vi "HostCameraManager.vi"() -> ()   [LabVIEW 2024]
panel:
  in  "Exposure":dbl(slide) scale=0.2..3.0
  out "Remote Capture":bool
  out "Live":bool
  out "FPS":dbl(graph)
  out "Image":u16[][](graph)
  in  "stop":bool
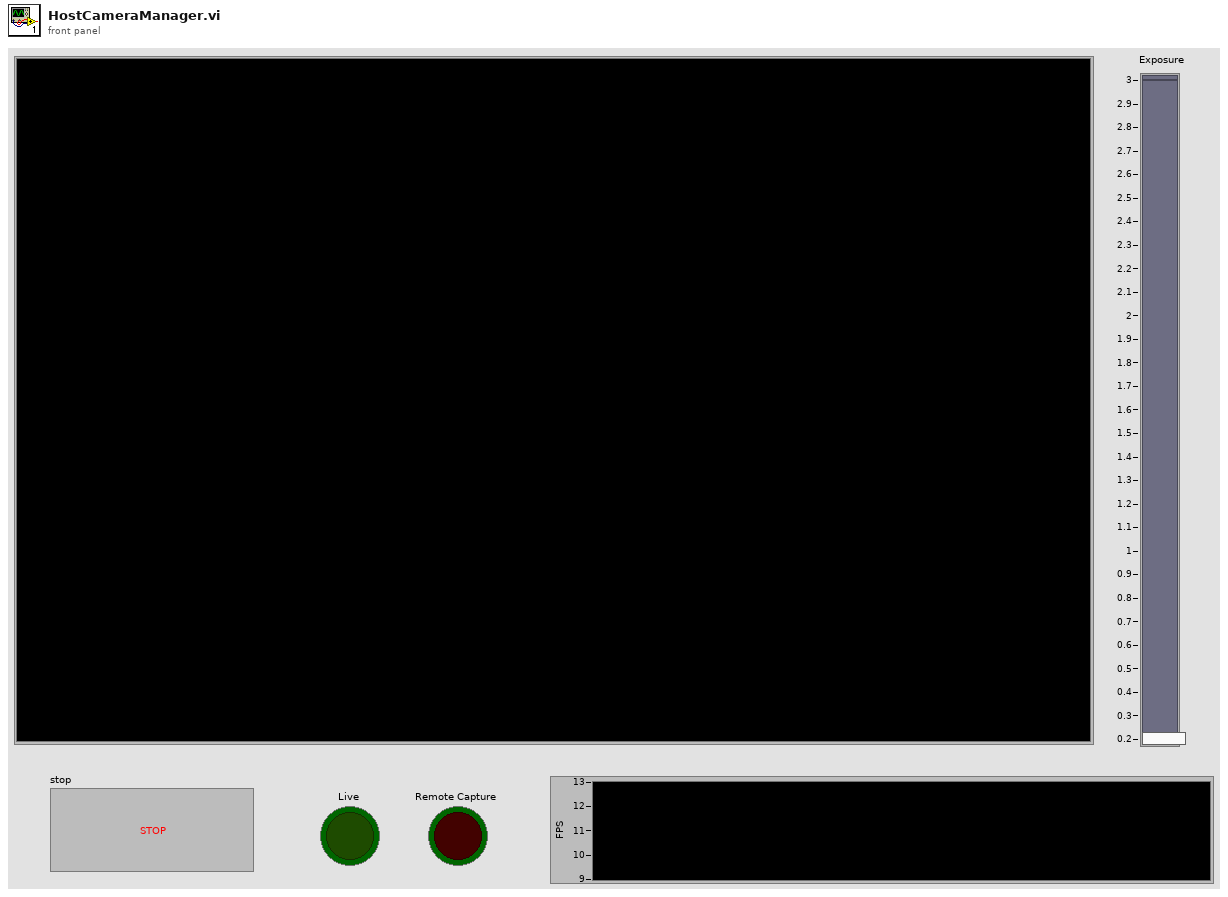
[diagram p1: front panel]
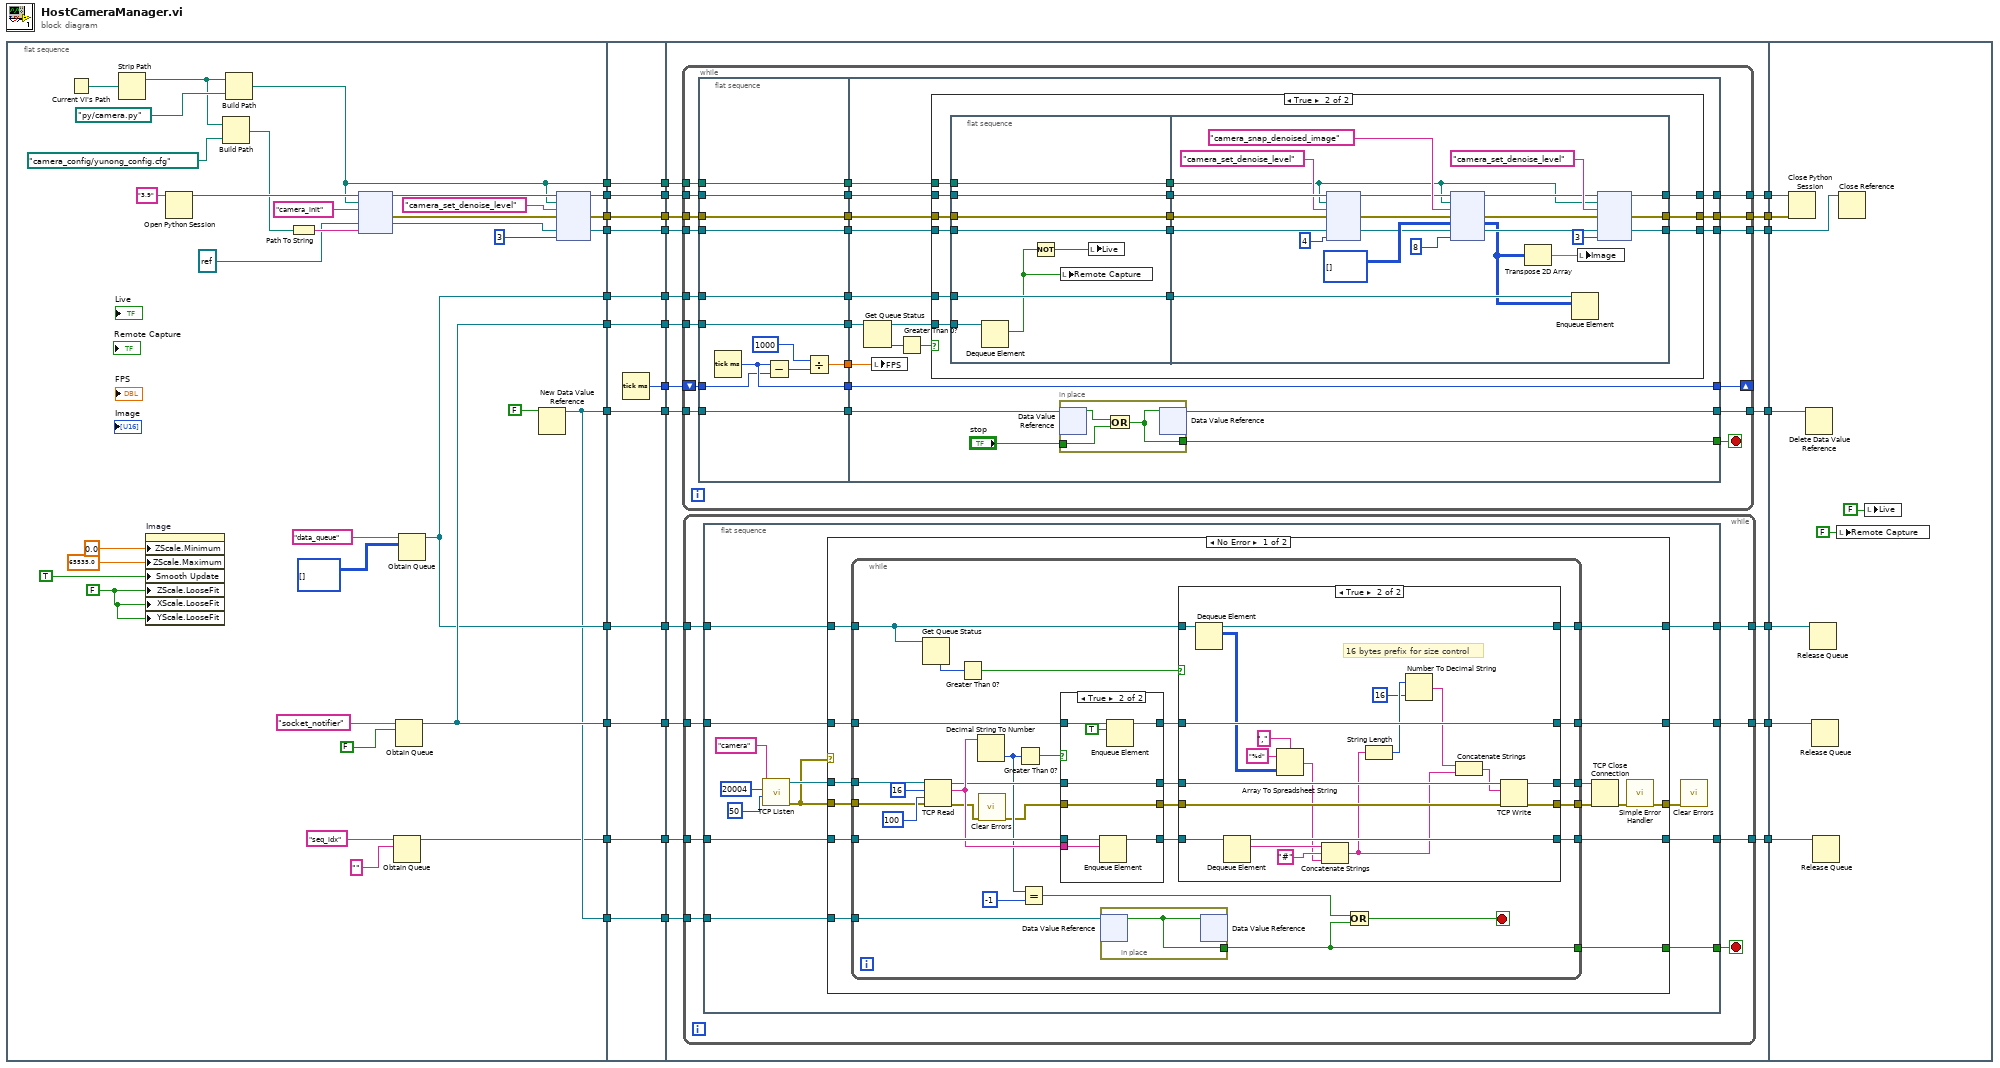
[diagram p0: block diagram]
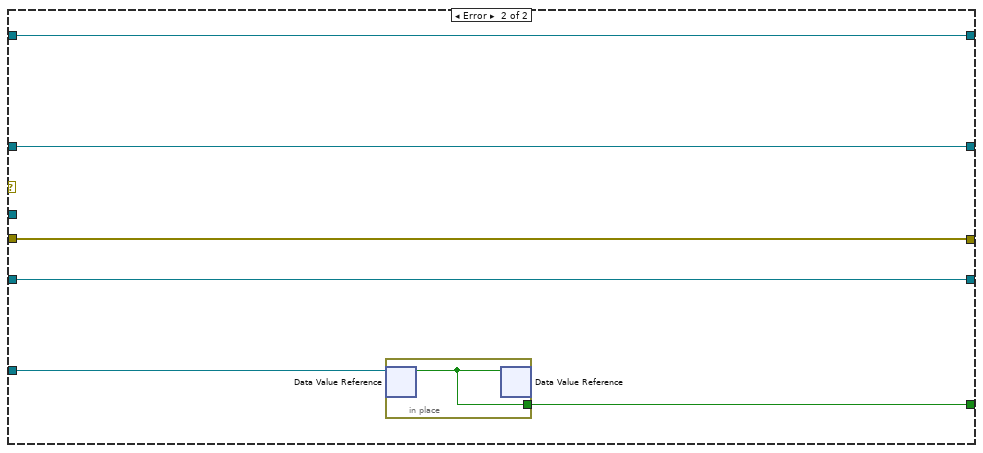
[diagram p4: hidden frame]
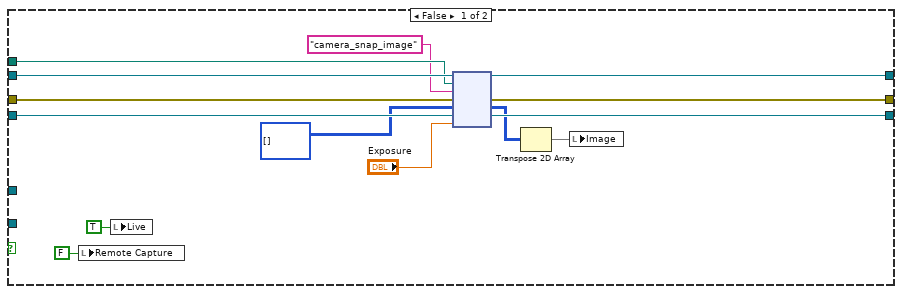
[diagram p5: hidden frame]
diagram:
  n1 = flat-sequence {
    tunnel: [w52] -> w27
    tunnel: [w51] -> w25
    tunnel: [w47] -> w23
    tunnel: [w46] -> w21
    tunnel: [w34] -> w17
    tunnel: [w36] -> w14
    tunnel: [w35] -> w12
    tunnel: [w36] -> w10
    tunnel: [w35] -> w8
    tunnel: [w34] -> w6
    tunnel: [w32] -> w4
    tunnel: w27 -> [w76]
    tunnel: [w76] -> w26
    tunnel: w25 -> [w75]
    tunnel: [w75] -> w24
    tunnel: w23 -> [w74]
    tunnel: [w74] -> w22
    tunnel: w21 -> [w73]
    tunnel: [w73] -> w20
    tunnel: [w72] -> w19
    tunnel: [w71] -> w18
    tunnel: w17 -> [w71]
    tunnel: [w70] -> w15
    tunnel: w14 -> [w70]
    tunnel: [w69] -> w13
    tunnel: w12 -> [w69]
    tunnel: [w68] -> w11
    tunnel: w10 -> [w68]
    tunnel: [w67] -> w9
    tunnel: w8 -> [w67]
    tunnel: [w66] -> w7
    tunnel: w6 -> [w66]
    tunnel: [w65] -> w5
    tunnel: w4 -> [w65]
    tunnel: w26 -> [w94]
    tunnel: w24 -> [w93]
    tunnel: w22 -> [w95]
    tunnel: w20 -> [w92]
    tunnel: [w91] -> w30
    tunnel: [w90] -> w29
    tunnel: [w89] -> w28
    tunnel: w19 -> [w88]
    tunnel: w18 -> [w87]
    tunnel: [w86] -> w16
    tunnel: w15 -> [w85]
    tunnel: w13 -> [w84]
    tunnel: w11 -> [w83]
    tunnel: w9 -> [w82]
    tunnel: w7 -> [w81]
    tunnel: w5 -> [w80]
    tunnel: [w79] -> w3
    tunnel: [w78] -> w2
    tunnel: [w77] -> w1
    tunnel: w30 -> [w329]
    tunnel: w29 -> [w328]
    tunnel: w28 -> [w327]
    tunnel: w16 -> [w326]
    tunnel: w3 -> [w325]
    tunnel: w2 -> [w324]
    tunnel: w1 -> [w323]
    frame #0 {
      w42 = FALSE ("Z Scale.Loose Fit")
      n2 = Current VI's Path() -> (path=w62:path)
      n3 = Strip Path(path=w62) -> (stripped path=w58:path)  [unwired: 1 out]
      n4 = property on="Image" class="IntGraph (strict)"("ZScale.Minimum"=0.0 ("Z Scale.Range:Minimum"), "ZScale.Maximum"=65535.0 ("Z Scale.Range:Maximum"), "Smooth Update"=TRUE, "ZScale.LooseFit"=w42, "XScale.LooseFit"=w42, "YScale.LooseFit"=w42) -> ()  [unwired: 2 in, 2 out]
      n5 = Open Python Session(python version="3.9" ("Python version")) -> (session out=w63:refnum<k35>)  [unwired: 2 in, 1 out]
      n6 = Build Path(base path=w58, name or relative path=path "camera_config/yunong_config.cfg") -> (appended path=w57:path)
      n7 = Build Path(base path=w58, name or relative path=path "py/camera.py") -> (appended path=w47:path)
      n8 = Path To String(path=w57) -> (string=w56:string)
      n9 = node(w63, w47, "camera_init" ("function name"), refnum<k38> refnum ("Python Object Refnum"), w56) -> (w55:refnum<k35>, w54:errorcluster, w49:refnum<k38>)  [unwired: 2 in, 2 out]
      n10 = Obtain Queue(name (unnamed)="seq_idx", element data type="" ("name (unnamed)")) -> (queue out=w32:refnum<queue>)  [unwired: 3 in, 2 out]
      n11 = Obtain Queue(name (unnamed)="socket_notifier", element data type=FALSE) -> (queue out=w36:refnum<queue>)  [unwired: 3 in, 2 out]
      n12 = Obtain Queue(name (unnamed)="data_queue", element data type=u16[][] []) -> (queue out=w35:refnum<queue>)  [unwired: 3 in, 2 out]
      n13 = New Data Value Reference(data value=FALSE) -> (data value reference=w34:refnum<data-value>)  [unwired: 1 in, 1 out]
      n14 = node(w55, w47, "camera_set_denoise_level" ("function name"), w54, w49, 3) -> (w52:refnum<k35>, w51:errorcluster, w46:refnum<k38>)  [unwired: 3 in, 2 out]
    }
    frame #1 {
      n15 = Tick Count (ms)() -> (millisecond timer value=w72:u32)
    }
    frame #2 {
      n16 = while {
        tunnel: w95 -> [w228]
        tunnel: w94 -> [w227]
        tunnel: w93 -> [w226]
        tunnel: w92 -> [w225]
        tunnel: [w224] -> w91
        tunnel: [w223] -> w90
        tunnel: [w222] -> w89
        shift-right: [w216] -> _
        shift-left: w88 -> [w214]
        tunnel: w87 -> [w213]
        tunnel: [w211] -> w86
        tunnel: w83 -> [w209]
        tunnel: w82 -> [w207]
        stop <- w210 stop-if-true
        n17 = flat-sequence {
          tunnel: w225 -> [w237]
          tunnel: w226 -> [w238]
          tunnel: w227 -> [w239]
          tunnel: w228 -> [w240]
          tunnel: [w240] -> w221
          tunnel: [w239] -> w220
          tunnel: [w238] -> w219
          tunnel: [w237] -> w218
          tunnel: [w236] -> w217
          tunnel: [w233] -> w215
          tunnel: w214 -> [w232]
          tunnel: w213 -> [w231]
          tunnel: [w231] -> w212
          tunnel: w209 -> [w230]
          tunnel: [w230] -> w208
          tunnel: w207 -> [w229]
          tunnel: [w229] -> w206
          tunnel: [w254] -> w224
          tunnel: [w253] -> w223
          tunnel: [w252] -> w222
          tunnel: w221 -> [w256]
          tunnel: w220 -> [w258]
          tunnel: w219 -> [w257]
          tunnel: w218 -> [w255]
          tunnel: [w251] -> w216
          tunnel: w217 -> [w251]
          tunnel: w215 -> [w250]
          tunnel: w212 -> [w249]
          tunnel: [w247] -> w211
          tunnel: [w246] -> w210
          tunnel: w208 -> [w245]
          tunnel: w206 -> [w241]
          frame #0 {
            n18 = Tick Count (ms)() -> (millisecond timer value=w236:u32)
            n19 = Subtract(x=w236, y=w232) -> (x-y=w235:u32)
            n20 = Divide(x=u32 1000, y=w235) -> (x/y=w233:dbl)
          }
          frame #1 {
            n21 = Get Queue Status(queue=w245) -> (queue out=w242:refnum<queue>, # elements in queue=w244:i32)  [unwired: 2 in, 6 out]
            n22 = local write "FPS"(w250) -> ()
            n23 = Greater Than 0?(x=w244) -> (x > 0?=w243:bool)
            n24 = case shown="True" w243 {
              tunnel: w258 -> [w272 w286]
              tunnel: w257 -> [w271 w285]
              tunnel: w256 -> [w270 w282]
              tunnel: w255 -> [w269 w284]
              tunnel: [w268 w283] -> w254
              tunnel: [w267 w281] -> w253
              tunnel: [w266 w280] -> w252
              tunnel: w242 -> [_ w273]
              tunnel: w241 -> [_ w279]
              frame False {
                n25 = local write "Remote Capture"(FALSE ("Remote Capture")) -> ()
                n26 = local write "Live"(TRUE ("Live")) -> ()
                n27 = node(w272, w270, "camera_snap_image" ("function name"), w271, u16[][] [], w269, "Exposure") -> (w268:refnum<k35>, w267:errorcluster, w263:u16[][], w266:refnum<k38>)  [unwired: 1 in, 2 out]
                n28 = Transpose 2D Array(2D array=w263) -> (transposed array=w262:u16[][])
                n29 = local write "Image"(w262) -> ()
              }
              frame True {
                n30 = flat-sequence {
                  tunnel: w279 -> [w290]
                  tunnel: w282 -> [w291]
                  tunnel: w284 -> [w292]
                  tunnel: w285 -> [w293]
                  tunnel: w286 -> [w294]
                  tunnel: [w294] -> w278
                  tunnel: [w293] -> w277
                  tunnel: [w292] -> w276
                  tunnel: [w291] -> w275
                  tunnel: [w290] -> w274
                  tunnel: w273 -> [w289]
                  tunnel: w278 -> [w317]
                  tunnel: w277 -> [w316]
                  tunnel: w276 -> [w314]
                  tunnel: w275 -> [w303]
                  tunnel: w274 -> [w298]
                  tunnel: [w306] -> w283
                  tunnel: [w300] -> w281
                  tunnel: [w299] -> w280
                  frame #0 {
                    n31 = Dequeue Element(queue=w289) -> (element=w288:bool)  [unwired: 2 in, 3 out]
                    n32 = Not(x=w288) -> (.not. x?=w287:bool)
                    n33 = local write "Remote Capture"(w288) -> ()
                    n34 = local write "Live"(w287) -> ()
                  }
                  frame #1 {
                    n35 = node(w317, w303, "camera_set_denoise_level" ("function name"), w316, w314, 4) -> (w310:refnum<k35>, w309:errorcluster, w302:refnum<k38>)  [unwired: 3 in, 2 out]
                    n36 = node(w310, w303, "camera_snap_denoised_image" ("function name"), w309, u16[][] [], w302, 8) -> (w305:refnum<k35>, w304:errorcluster, w297:u16[][], w301:refnum<k38>)  [unwired: 1 in, 2 out]
                    n37 = Transpose 2D Array(2D array=w297) -> (transposed array=w296:u16[][])
                    n38 = Enqueue Element(queue=w298, element=w297) -> ()  [unwired: 2 in, 3 out]
                    n39 = local write "Image"(w296) -> ()
                    n40 = node(w305, w303, "camera_set_denoise_level" ("function name"), w304, w301, 3) -> (w306:refnum<k35>, w300:errorcluster, w299:refnum<k38>)  [unwired: 3 in, 2 out]
                  }
                }
              }
            }
            n41 = in-place {
              in-place-border: "stop" -> [w319]
              in-place-border: [w318] -> w246
              n42 = in-place-dvr #1(w249) -> (w320:bool)  [unwired: 1 out]
              n43 = Or(x=w320, y=w319) -> (x .or. y?=w318:bool)
              n44 = in-place-dvr #1(w318) -> (w247:refnum<data-value>)  [unwired: 1 out]
            }
          }
        }
      }
      n45 = while {
        tunnel: w85 -> [w103]
        tunnel: w84 -> [w102]
        tunnel: w81 -> [w101]
        tunnel: w80 -> [w100]
        tunnel: [w98] -> w79
        tunnel: [w97] -> w78
        tunnel: [w96] -> w77
        stop <- w99 stop-if-true
        n46 = flat-sequence {
          tunnel: w102 -> [w115]
          tunnel: w103 -> [w114]
          tunnel: w101 -> [w110]
          tunnel: w100 -> [w107]
          tunnel: [w112] -> w98
          tunnel: [w111] -> w96
          tunnel: [w109] -> w97
          tunnel: [w108] -> w99
          frame #0 {
            n47 = call <vilib>:"TCP Listen.vi"("timeout ms (wait forever: -1)"=50, "port"=u16 20004, "service name"="camera") -> ("error out"=w104:errorcluster, "connection ID"=w113:refnum<k5>)  [unwired: 4 in, 3 out]
            n48 = case shown="No Error" w104 {
              tunnel: w115 -> [w131 w203]
              tunnel: w114 -> [w130 w202]
              tunnel: w113 -> [w129 _]
              tunnel: w107 -> [w128 w204]
              tunnel: [w127 w203] -> w112
              tunnel: [w126 w204] -> w111
              tunnel: w110 -> [w125 w201]
              tunnel: w104 -> [w124 w199]
              tunnel: [w123 w202] -> w109
              tunnel: [w122 w200] -> w108
              tunnel: [w118 w199] -> w106
              frame No Error {
                n49 = while {
                  tunnel: w130 -> [w157]
                  tunnel: w129 -> [w156]
                  tunnel: w125 -> [w141]
                  tunnel: w124 -> [w150]
                  tunnel: w128 -> [w148]
                  tunnel: [w153] -> w126
                  tunnel: [w142] -> w123
                  tunnel: w131 -> [w159]
                  tunnel: [w154] -> w127
                  tunnel: [w134] -> w122
                  tunnel: [w140] -> w121
                  tunnel: [w139] -> w120
                  stop <- w135 stop-if-true
                  n50 = Get Queue Status(queue=w159) -> (# elements in queue=w160:i32)  [unwired: 2 in, 7 out]
                  n51 = TCP Read(connection ID=w156, bytes to read=16, error in (no error)=w150, 9:100 ("timeout ms (25000)")) -> (connection ID out=w145:refnum<k5>, data out=w147:string, error out=w133:errorcluster)  [unwired: 1 in]
                  n52 = Greater Than 0?(x=w160) -> (x > 0?=w158:bool)
                  n53 = Decimal String To Number(string=w147) -> (number=w138:i32)  [unwired: 2 in, 1 out]
                  n54 = call <vilib>:"Clear Errors.vi"("error in (no error)"=w133) -> ("error out"=w132:errorcluster)  [unwired: 5 in, 1 out]
                  n55 = Greater Than 0?(x=w138) -> (x > 0?=w149:bool)
                  n56 = Equal?(x=w138, y=-1) -> (x = y?=w136:bool)
                  n57 = case shown="True" w149 {
                    tunnel: w157 -> [w165 w173]
                    tunnel: [w165 w172] -> w155
                    tunnel: w148 -> [w164 w170]
                    tunnel: w147 -> [_ w169]
                    tunnel: [w164 w168] -> w146
                    tunnel: w145 -> [w163 w167]
                    tunnel: w132 -> [w162 w166]
                    tunnel: [w163 w167] -> w144
                    tunnel: [w162 w166] -> w143
                    frame False {
                    }
                    frame True {
                      n58 = Enqueue Element(queue=w170, element=w169) -> (queue out=w168:refnum<queue>)  [unwired: 2 in, 2 out]
                      n59 = Enqueue Element(queue=w173, element=TRUE) -> (queue out=w172:refnum<queue>)  [unwired: 2 in, 2 out]
                    }
                  }
                  n60 = in-place {
                    in-place-border: [w161] -> w134
                    n61 = in-place-dvr #2(w141) -> (w161:bool)  [unwired: 1 out]
                    n62 = in-place-dvr #2(w161) -> ()  [unwired: 2 out]
                  }
                  n63 = case shown="True" w158 {
                    tunnel: w159 -> [w178 w198]
                    tunnel: w146 -> [w177 w196]
                    tunnel: w155 -> [w176 w192]
                    tunnel: [w178 w197] -> w154
                    tunnel: [w177 w194] -> w153
                    tunnel: w144 -> [w175 w191]
                    tunnel: w143 -> [w174 w190]
                    tunnel: [w176 w192] -> w142
                    tunnel: [w175 w185] -> w140
                    tunnel: [w174 w184] -> w139
                    frame False {
                    }
                    frame True {
                      # "16 bytes prefix for size control"
                      n64 = Dequeue Element(queue=w198) -> (queue out=w197:refnum<queue>, element=w189:u16[][])  [unwired: 2 in, 2 out]
                      n65 = Dequeue Element(queue=w196) -> (queue out=w194:refnum<queue>, element=w195:string)  [unwired: 2 in, 2 out]
                      n66 = Array To Spreadsheet String(delimiter (Tab)=",", array=w189, 3:"%d" ("format string")) -> (spreadsheet string=w186:string)
                      n67 = Concatenate Strings(w195, "#" ("string"), w186) -> (w181:string)
                      n68 = String Length(string=w181) -> (length=w183:i32)
                      n69 = Number To Decimal String(number=w183, width (-)=i16 16) -> (decimal integer string=w180:string)
                      n70 = Concatenate Strings(w180, w181) -> (w179:string)
                      n71 = TCP Write(connection ID=w191, data in=w179, error in (no error)=w190) -> (connection ID out=w185:refnum<k5>, error out=w184:errorcluster)  [unwired: 1 in, 1 out]
                    }
                  }
                  n72 = Or(x=w136, y=w134) -> (x .or. y?=w135:bool)
                }
                n73 = TCP Close Connection(connection ID=w121, error in (no error)=w120) -> (error out=w119:errorcluster)  [unwired: 1 in, 1 out]
                n74 = call <vilib>:"Simple Error Handler.vi"("error in (no error)"=w119) -> ("error out"=w118:errorcluster)  [unwired: 4 in, 4 out]
              }
              frame Error {
                n75 = in-place {
                  in-place-border: [w205] -> w200
                  n76 = in-place-dvr #3(w201) -> (w205:bool)  [unwired: 1 out]
                  n77 = in-place-dvr #3(w205) -> ()  [unwired: 2 out]
                }
              }
            }
            n78 = call <vilib>:"Clear Errors.vi"("error in (no error)"=w106) -> ()  [unwired: 5 in, 2 out]
          }
        }
      }
    }
    frame #3 {
      n79 = Close Python Session(session in=w329, error in=w328) -> ()  [unwired: 1 out]
      n80 = Delete Data Value Reference(data value reference=w326) -> ()  [unwired: 1 in, 2 out]
      n81 = Release Queue(queue=w325) -> ()  [unwired: 2 in, 3 out]
      n82 = Release Queue(queue=w324) -> ()  [unwired: 2 in, 3 out]
      n83 = Release Queue(queue=w323) -> ()  [unwired: 2 in, 3 out]
      n84 = local write "Remote Capture"(FALSE ("Remote Capture")) -> ()
      n85 = Close Reference(reference=w327) -> ()  [unwired: 1 in, 1 out]
      n86 = local write "Live"(FALSE ("Live")) -> ()
    }
  }
